vi "Cull and Group.vi"(6 "Line Border":cluster{"Top":dbl, "Bottom":dbl}={"Top"=6.0, "Bottom"=1.0}, 9 "Score Cutoff":dbl=3.0, 10 "Sorted Data":dbl[][](array[numeric])) -> (0 "Rect":T1, 1 "Line":T1, 2 "Score":dbl, 3 "Center":cluster{"X":dbl, "Y":dbl})   [LabVIEW 2016]
doc: "Examine the particle measurements to find the most likely pair that make up the target. This mostly compares the edges of the bounding boxes. It then returns information about the overall target, notably the rectangle sourrounding the particles, the vertical line that bisects the target, and the center of the top particle."
panel:
  out "Grouping Scores":T2(array[cluster])
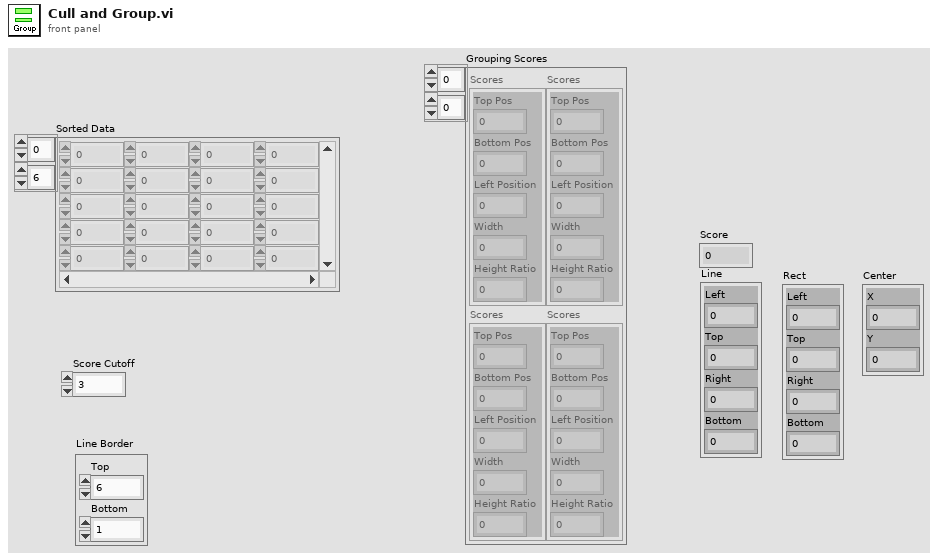
[diagram p1: front panel]
types:
  T1 = cluster{"Left":dbl, "Top":dbl, "Right":dbl, "Bottom":dbl}
  T2 = cluster{"Top Pos":dbl, "Bottom Pos":dbl, "Left Position":dbl, "Width":dbl, "Height Ratio":dbl}[][]
  T3 = cluster{"Top Position":dbl, "Bottom Position":dbl, "Left Gap":dbl, "Width":dbl, "Height Ratio":dbl}
  T4 = cluster{"Left":dbl, "Numeric":dbl, "Right":dbl, "Numeric":dbl}
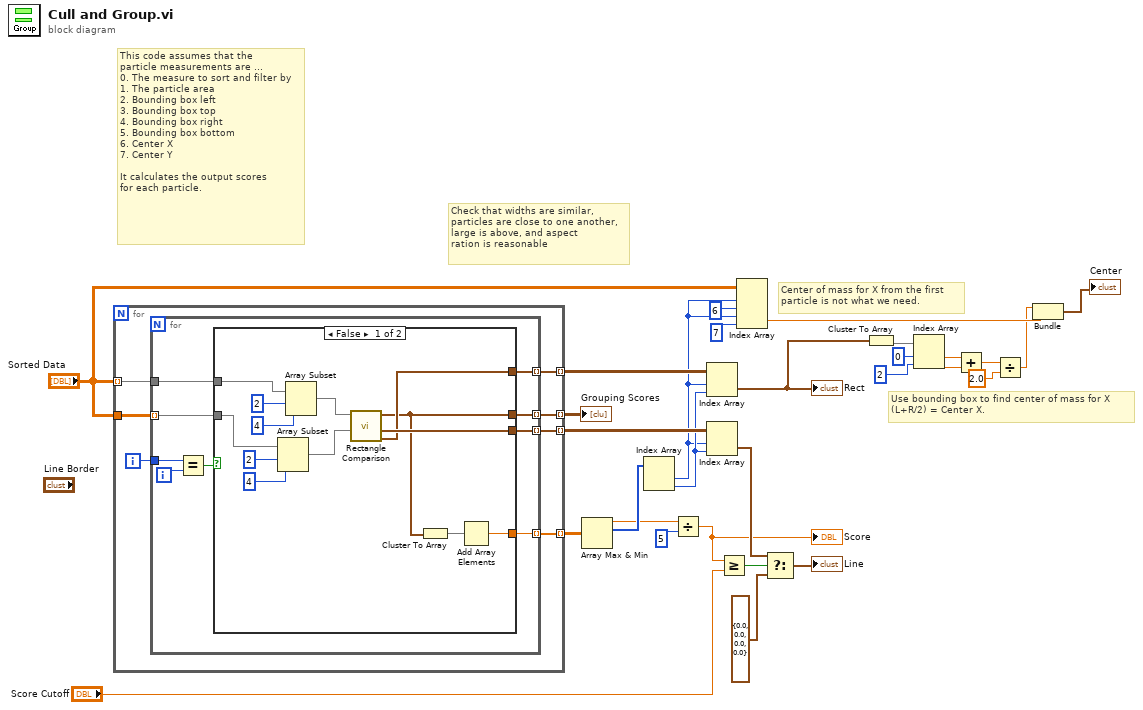
[diagram p0: block diagram]
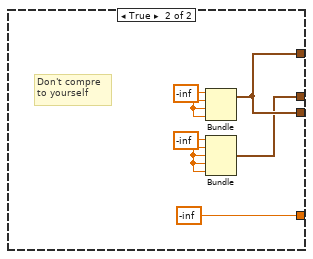
[diagram p2: hidden frame]
diagram:
  # "Center of mass for X from the first \nparticle is not what we need."
  # "Use bounding box to find center of mass for X\n(L+R/2) = Center X."
  # "Check that widths are similar,\nparticles are close to one another,\nlarge is above, and aspect\nration is reasonable"
  # "This code assumes that the\nparticle measurements are ...\n0. The measure to sort and filter by\n1. The particle area\n2. Bounding box left\n3. Bounding box top\n4. Bounding box right\n5. Bounding box bottom\n6. Center X\n7. Center Y\n\nIt calculates the output scores\nfor each particle."
  n1 = for {
    tunnel: "Sorted Data" -> [w36] mode=indexing
    tunnel: "Sorted Data" -> [w35]
    tunnel: [w34] -> w29 mode=indexing
    tunnel: [w32] -> w28 mode=indexing
    tunnel: [w31] -> w25 mode=indexing
    tunnel: [w30] -> w21 mode=indexing
    i -> [w33]
    n2 = for {
      tunnel: w36 -> [w45]
      tunnel: w35 -> [w43] mode=indexing
      tunnel: [w42] -> w34 mode=indexing
      tunnel: w33 -> [w41]
      tunnel: [w39] -> w32 mode=indexing
      tunnel: [w38] -> w31 mode=indexing
      tunnel: [w37] -> w30 mode=indexing
      i -> [w40]
      n3 = Equal?(x=w41, y=w40) -> (x = y?=w44:bool)
      n4 = case shown="False" w44 {
        tunnel: w45 -> [w56 _]
        tunnel: w43 -> [w53 _]
        tunnel: [w46 w59] -> w42
        tunnel: [w51 -inf] -> w39
        tunnel: [w48 w62] -> w38
        tunnel: [w47 w62] -> w37
        frame False {
          n5 = Array Subset(array=w53, index=2, length=4) -> (w49:dbl[])
          n6 = Array Subset(array=w56, index=2, length=4) -> (w50:dbl[])
          n7 = call "Rectangle Comparison.vi"("Second"=w49, "First"=w50) -> ("Rect"=w47:T1, "Line"=w48:T1, "Scores"=w46:T3)  [unwired: 7 in]
          n8 = Cluster To Array(cluster=w46) -> (array=w52:dbl[])
          n9 = Add Array Elements(numeric array=w52) -> (sum=w51:dbl)
        }
        frame True {
          w60 = -inf
          w61 = -inf
          # "Don't compre\nto yourself"
          n10 = Bundle(w61, w61, w61, w61) -> (w62:cluster{dbl, dbl, dbl, dbl})  [unwired: 1 in]
          n11 = Bundle(w60, w60, w60, w60, w60) -> (w59:cluster{dbl, dbl, dbl, dbl, dbl})  [unwired: 1 in]
        }
      }
    }
  }
  "Grouping Scores" <- w29
  n12 = Array Max & Min(array=w28) -> (max value=w12:dbl, max index (indices)=w13:i32[])  [unwired: 2 out]
  n13 = Index Array(array=w13) -> (element #1=w18:i32, element #2=w20:i32)  [unwired: 2 in]
  n14 = Divide(x=w12, y=5 ("length")) -> (x/y=w11:dbl)
  "Score" <- w11
  n15 = Index Array(array=w21, index (row)=w18, index (col)=w20) -> (element=w9:T1)
  "Rect" <- w9
  n16 = Index Array(array=w25, index (row)=w18, index (col)=w20) -> (element=w24:T1)
  n17 = Greater Or Equal?(x=w11, y="Score Cutoff") -> (x >= y?=w27:bool)
  n18 = Index Array(array="Sorted Data", index (row) #1=w18, index (col) #1=6 ("index"), index (row) #2=w18, index (col) #2=7 ("index")) -> (element #2=w16:dbl)  [unwired: 1 out]
  n19 = Select(t=w24, s=w27, f=cluster{dbl, "Numeric":dbl, dbl, "Numeric":dbl} {0.0, "Numeric"=0.0, 0.0, "Numeric"=0.0}) -> (s? t:f=→"Line":T4)
  n20 = Cluster To Array(cluster=w9) -> (array=w8:dbl[])
  n21 = Index Array(array=w8, index #1=0 ("index"), index #2=2 ("index")) -> (element #1=w5:dbl, element #2=w4:dbl)
  n22 = Add(x=w5, y=w4) -> (x+y=w3:dbl)
  n23 = Divide(x=w3, y=2.0) -> (x/y=w1:dbl)
  n24 = Bundle(w1, "Numeric"=w16) -> (→"Center":cluster{dbl, "Numeric":dbl})  [unwired: 1 in]
